vi "InstrParam.vi"(4 "queue out":refnum<queue>, 6 "user event out":refnum<user-event>, 8 "error in (no error)":errorcluster caption="entrée d'erreur (pas d'erreur)", 10 "InstrParam":string, 11 "SR400 en entrée":refnum<class "DK240.lvclass"> caption="DNL_LabVIEW Object in") -> (0 "error out":errorcluster caption="sortie d'erreur", 3 "SR400 en sortie":refnum<class "DK240.lvclass"> caption="DNL_LabVIEW Object out")   [LabVIEW 2019, in "DK240.lvclass"]
uses:
  DK240.lvclass
  C:/Programmes Labview/LabScanV1A/DevicesClass/BaseDevice/BaseDevice.lvclass
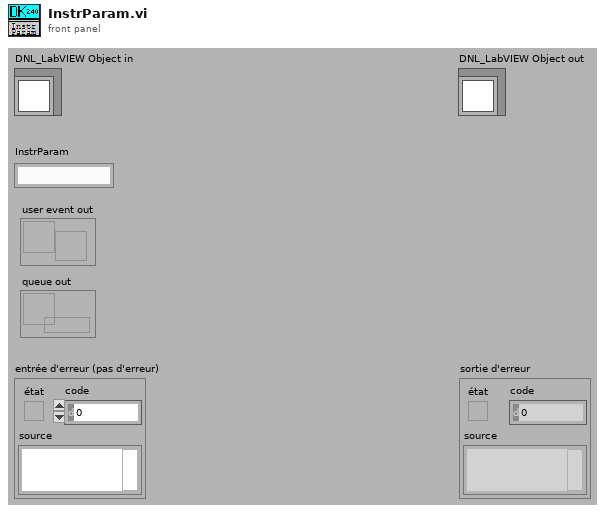
[diagram p1: front panel]
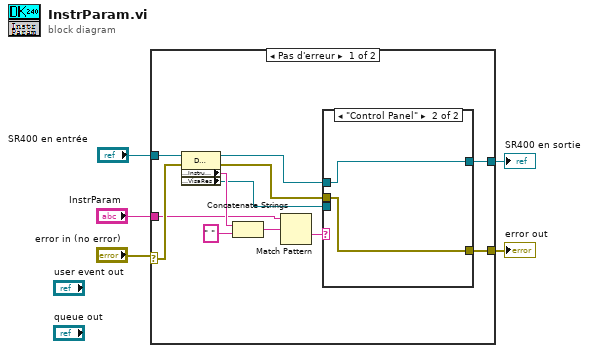
[diagram p0: block diagram]
diagram:
  n1 = case shown="Pas d'erreur" "error in (no error)" {
    selector: "error in (no error)" -> [w16 w22]
    tunnel: "SR400 en entrée" -> [w17 w23]
    tunnel: [w12 w23] -> w3
    tunnel: [w9 w22] -> w2
    tunnel: "InstrParam" -> [w6 _]
    frame No Error {
      n2 = property class="DK240.lvclass"(reference=w17, error in=w16) -> (reference out=w11:refnum<class "DK240.lvclass">, error out=w10:errorcluster, "Accessor:InstrumentName"=w14:string, "Accessor:VisaRes"=w8:refnum<visa-resource-name>)
      n3 = Concatenate Strings(w14, " " ("chaîne")) -> (w7:string)
      n4 = Match Pattern(string=w6, regular expression=w7) -> (after substring=w13:string)  [unwired: 1 in, 3 out]
      n5 = case shown="\"Control Panel\"" w13 {
        tunnel: [w19 w21] -> w12
        tunnel: w11 -> [w19 w21]
        tunnel: w10 -> [w18 w20]
        tunnel: [w18 w20] -> w9
        tunnel: w8 -> [_ _]
        frame Default {
        }
        frame "Control Panel" {
        }
      }
    }
    frame Error {
    }
  }
  "error out" <- w2
  "SR400 en sortie" <- w3
